vi "Initialize.vi"(8 "error in (no error)":errorcluster, 11 "Instrument Detection in":refnum<class "Instrument Detection.lvclass">) -> (0 "error out":errorcluster, 3 "Instrument Detection out":refnum<class "Instrument Detection.lvclass">)   [LabVIEW 2020, in "Instrument Detection.lvlib" / "Instrument Detection.lvclass"]
doc: "Initialize the Instrument Detection class."
uses:
  Instrument Detection.lvclass
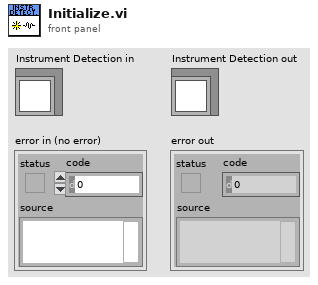
[diagram p1: front panel]
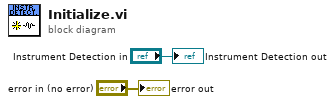
[diagram p0: block diagram]
diagram:
  "error out" <- "error in (no error)"
  "Instrument Detection out" <- "Instrument Detection in"
